vi "Project Path Getter.vi"(11 "error in (no error)":errorcluster) -> (4 "Path":path, 15 "error out":errorcluster)   [LabVIEW 2021, in "Dictionary.lvlib"]
uses:
  Dictionary.lvlib
  controls/Dictionary States.ctl
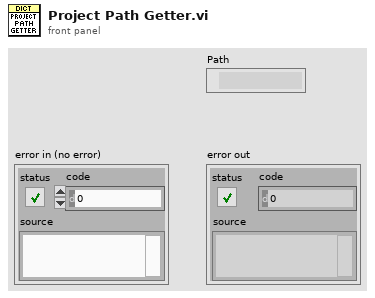
[diagram p1: front panel]
types:
  T1 = typedef "Dictionary.lvlib/Dictionary States.ctl" = enum16{"Set", "Get", "Delete", "Delete All"}
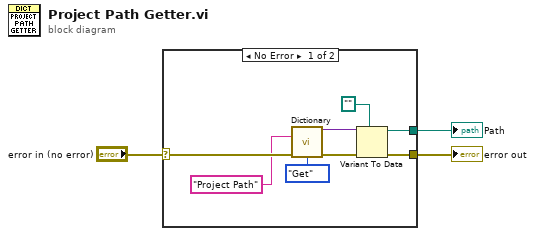
[diagram p0: block diagram]
diagram:
  n1 = case shown="No Error" "error in (no error)" {
    selector: "error in (no error)" -> [w9 w12]
    tunnel: [w7 w12] -> w2
    tunnel: [w6 _] -> w1
    frame No Error {
      n2 = call "Dictionary.vi"("Key"="Project Path", "error in (no error)"=w9, "Dictionary States"=Dictionary_States."Get" ("Dict States")) -> ("Variant_Out"=w5:variant, "error out"=w8:errorcluster)  [unwired: 11 in]
      n3 = Variant To Data(error in=w8, type=path "", Variant=w5) -> (data=w6:path, error out=w7:errorcluster)
    }
    frame Error {
    }
  }
  "error out" <- w2
  "Path" <- w1
